vi "Find All Highlights.vi"(11 "String":string) -> (3 "Sections":T1(array[cluster]))   [LabVIEW 2020]
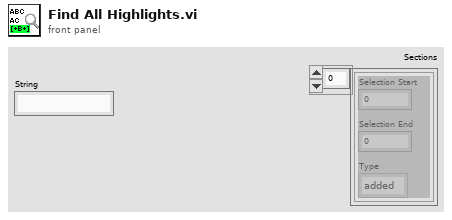
[diagram p1: front panel]
types:
  T1 = cluster{"Selection Start":u32, "Selection End":u32, "Type":enum16{"added", "missing"}}[]
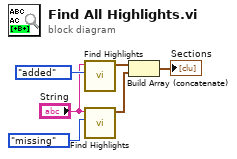
[diagram p0: block diagram]
diagram:
  n1 = call "Find Highlights.vi"("Type"=enum16{"added", "missing"}."added", "String"="String") -> ("Sections"=w4:T1)  [unwired: 9 in]
  n2 = call "Find Highlights.vi"("Type"=enum16{"added", "missing"}."missing", "String"="String") -> ("Sections"=w1:T1)  [unwired: 9 in]
  n3 = Build Array (concatenate)(w4, w1) -> (→"Sections":T1)
